vi "Get BLISS_Log Changed Controls.vi"(9 "Data Parameters":T1) -> (3 "Data Parameters out":T1)   [LabVIEW 2020]
uses:
  MC5e Squad_Info.ctl
  MC5e Unit_Status_List.ctl
  MC5e Data_Parameters.ctl
  MC5e Terrain types.ctl
  Location.ctl
  MC5e Unit.ctl
  MC5e Force.ctl
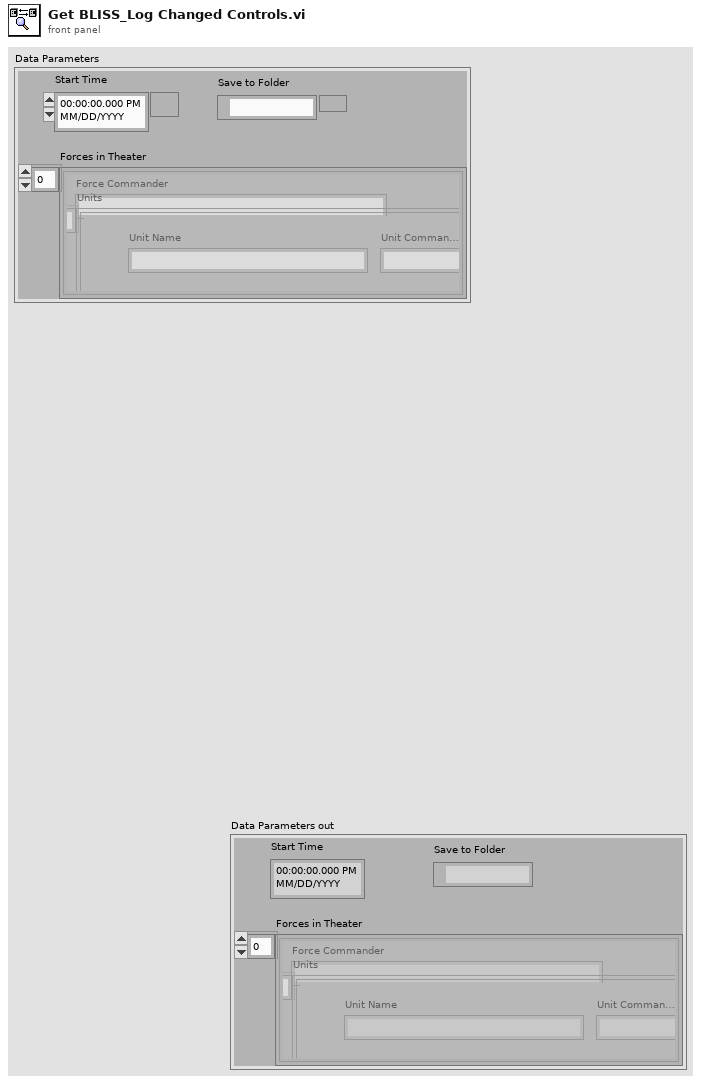
[diagram p1: front panel]
types:
  T1 = typedef "MC5e Data_Parameters.ctl" = cluster{"Start Time":timestamp, "Save to Folder":path, "Forces in Theater":T2[]}
  T2 = typedef "MC5e Force.ctl" = cluster{"Force Commander":string, "Units":T3[]}
  T3 = typedef "MC5e Unit.ctl" = cluster{"Squad List":T4, "Unit Fatigue Level":enum16{"Not Fatigued", "Fatigued", "Seriously Fatigued"}, "Flying Unit":bool, "Mounted Unit":bool, "Difficult Terrain Types":T6, "Full BR":dbl, "Defending from Stronghold":bool, "Speed":dbl, "Capacity %":dbl, "Morale":dbl, "Current BR":dbl, "Location":T7, "Unit Name":string, "Unit Commander":string, "Unit Notes":string}
  T4 = typedef "MC5e Unit_Status_List.ctl" = T5[]
  T5 = typedef "MC5e Squad_Info.ctl" = cluster{"Squad Name":string, "# Soldiers":dbl, "Battle Rating":dbl, "Flying":bool, "Mounted":bool, "Speed":dbl, "Range":dbl, "Morale":dbl, "Token Image":variant, "Max Endurance":dbl, "Current Endurance":dbl, "Difficult Terrain":T6}
  T6 = typedef "MC5e Terrain types.ctl" = cluster{"Artic / snow / ice)":bool, "Coast":bool, "Desert / sand":bool, "Forest / woodland":bool, "Grassland / plains":bool, "Mountain / canyons":bool, "Underdark / caverns":bool, "Acquatic / rivers, lakes, ocean":bool}
  T7 = typedef "Location.ctl" = cluster{"X coordinate":dbl, "Y coordinate":dbl}
  T8 = enum16{"Get Only Reject Images", "Get Only PBQA Images", "Get Both PBQA And Reject Images"}
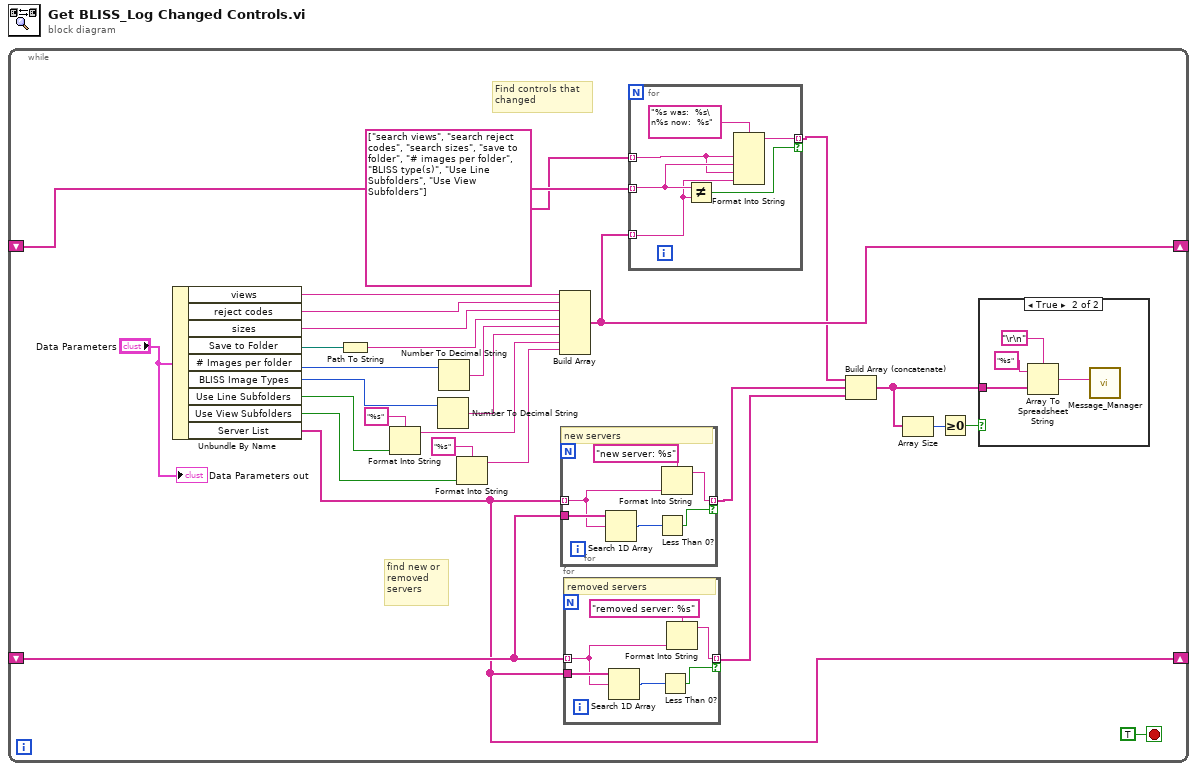
[diagram p0: block diagram]
diagram:
  n1 = while {
    shift-right: [w17] -> _
    shift-left: _ -> [w16]
    shift-right: [w3] -> _
    shift-left: _ -> [w14]
    stop <- TRUE stop-if-true
    # "find new or\nremoved \nservers"
    # "Find controls that \nchanged"
    n2 = Unbundle By Name("Data Parameters") -> ("views"=w24:string, "reject codes"=w23:string, "sizes"=w22:string, "Save to Folder"=w21:path, "# Images per folder"=w26:i32, "BLISS Image Types"=w25:T8, "Use Line Subfolders"=w6:bool, "Use View Subfolders"=w2:bool, "Server List"=w3:string[])
    n3 = Path To String(path=w21) -> (string=w20:string)
    n4 = Format Into String(format string="%s", w6) -> (resulting string=w5:string)  [unwired: 2 in, 1 out]
    n5 = Number To Decimal String(number=w25) -> (decimal integer string=w18:string)  [unwired: 1 in]
    n6 = Number To Decimal String(number=w26) -> (decimal integer string=w19:string)  [unwired: 1 in]
    n7 = Format Into String(format string="%s", w2) -> (resulting string=w1:string)  [unwired: 2 in, 1 out]
    n8 = Build Array(w24, w23, w22, w20, w19, w18, w5, w1) -> (w17:string[])
    n9 = for {
      tunnel: w3 -> [w40] mode=indexing
      tunnel: w14 -> [w44]
      tunnel: [w39] -> w12 mode=indexing if=w42
      # "new servers"
      n10 = Search 1D Array(1D array=w44, element=w40) -> (index of element=w43:i32)  [unwired: 1 in]
      n11 = Less Than 0?(x=w43) -> (x < 0?=w42:bool)
      n12 = Format Into String(format string="new server: %s", w40) -> (resulting string=w39:string)  [unwired: 2 in, 1 out]
    }
    n13 = for {
      tunnel: w14 -> [w34] mode=indexing
      tunnel: w3 -> [w38]
      tunnel: [w33] -> w11 mode=indexing if=w36
      # "removed servers"
      n14 = Search 1D Array(1D array=w38, element=w34) -> (index of element=w37:i32)  [unwired: 1 in]
      n15 = Less Than 0?(x=w37) -> (x < 0?=w36:bool)
      n16 = Format Into String(format string="removed server: %s", w34) -> (resulting string=w33:string)  [unwired: 2 in, 1 out]
    }
    n17 = for {
      tunnel: w17 -> [w47] mode=indexing
      tunnel: w16 -> [w49] mode=indexing
      tunnel: string[] ["search views", "search reject codes", "search sizes", "save to folder", "# images per folder", "BLISS type(s)", "Use Line Subfolders", "Use View Subfolders"] -> [w48] mode=indexing
      tunnel: [w46] -> w13 mode=indexing if=w45
      n18 = Not Equal?(x=w49, y=w47) -> (x != y?=w45:bool)
      n19 = Format Into String(format string="%s was:  %s\n%s now:  %s", w48, w49, w48, w47) -> (resulting string=w46:string)  [unwired: 2 in, 1 out]
    }
    n20 = Build Array (concatenate)(w13, w12, w11) -> (w10:string[])
    n21 = Array Size(array=w10) -> (size(s)=w9:i32)
    n22 = Greater Or Equal To 0?(x=w9) -> (x >= 0?=w8:bool)
    n23 = case shown="True" w8 {
      tunnel: w10 -> [_ w30]
      frame False {
      }
      frame True {
        n24 = Array To Spreadsheet String(delimiter (Tab)="\r\n", array=w30, 3:"%s" ("format string")) -> (spreadsheet string=w29:string)
        n25 = call "Message_Manager.vi"("New Entry"=w29) -> ()  [unwired: 5 in, 6 out]
      }
    }
    "Data Parameters out" <- "Data Parameters"
  }
